vi "WILT Index Station Stats.vi"(0 "Station Number":u32, 1 "Cool Down Period (seconds)":dbl[](array[numeric]), 2 "Drying Time (Min)":dbl[](array[numeric]), 3 "Previous Run Statistics":T1[](array[typedef]), 4 "Enable Start Retry in":bool[](array[boolean]), 5 "Error In":errorcluster) -> (14 "Station Array Index":u32, 15 "Station Cool Down Period (Sec)":dbl, 16 "Station Drying Time (Min)":dbl, 17 "Previous Cycle Time (Minutes)":dbl, 18 "Enable Start Retry out":bool, 19 "Error Out":errorcluster)   [LabVIEW 2016]
uses:
  Type Definitions/WILT Summary Data.ctl
panel:
  # "Get The Info Associated with the desired station"
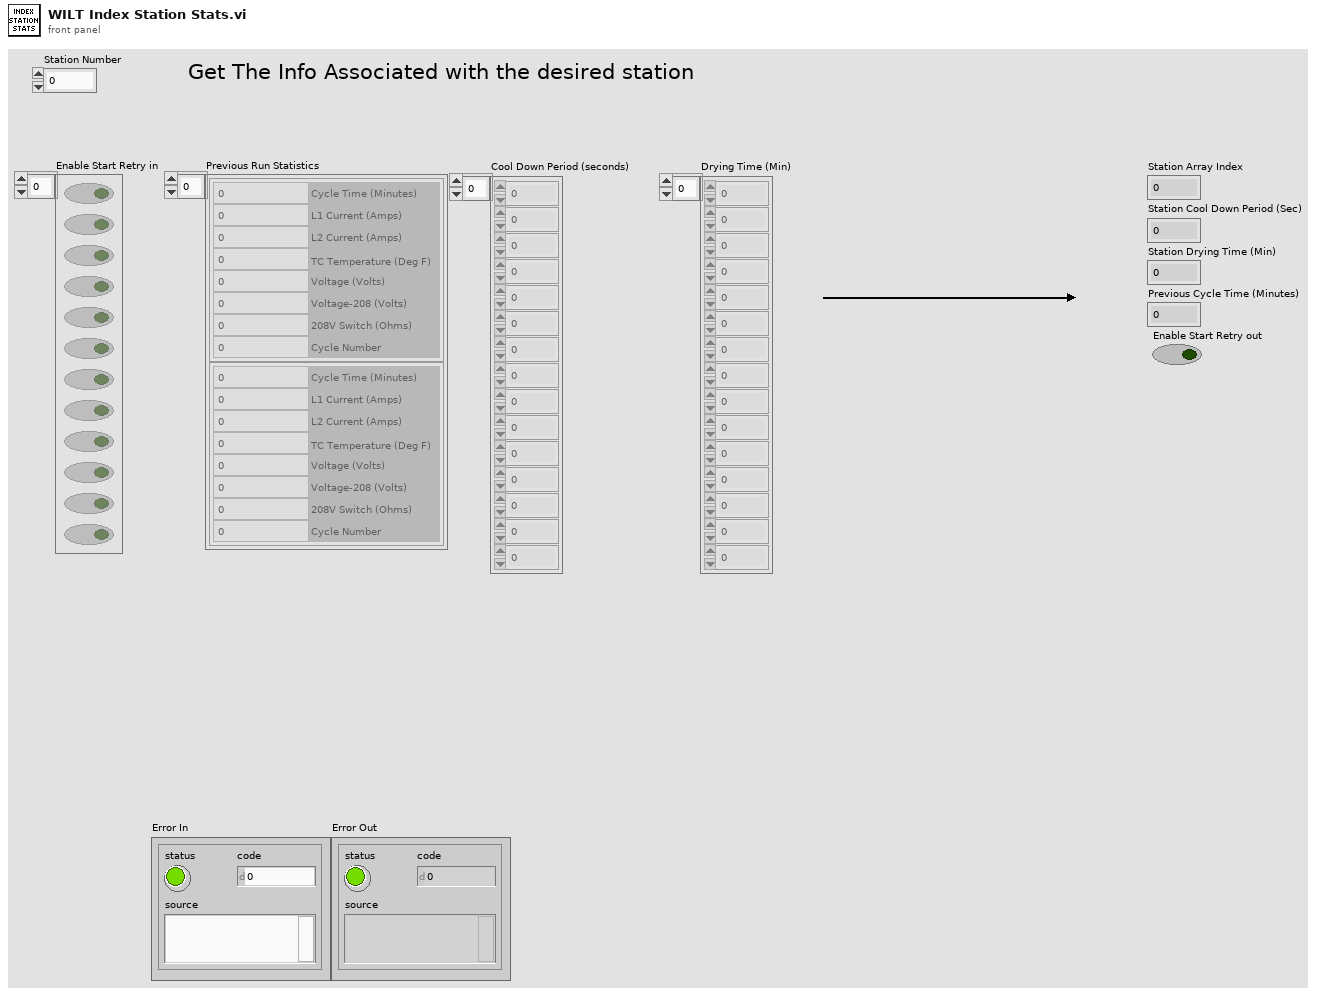
[diagram p1: front panel]
types:
  T1 = typedef "WILT Summary Data.ctl" = cluster{"Cycle Time (Minutes)":dbl, "L1 Current (Amps)":dbl, "L2 Current (Amps)":dbl, "TC Temperature (Deg F)":dbl, "Voltage (Volts)":dbl, "Voltage-208 (Volts)":dbl, "208V Switch (Ohms)":dbl, "Cycle Number":i32}
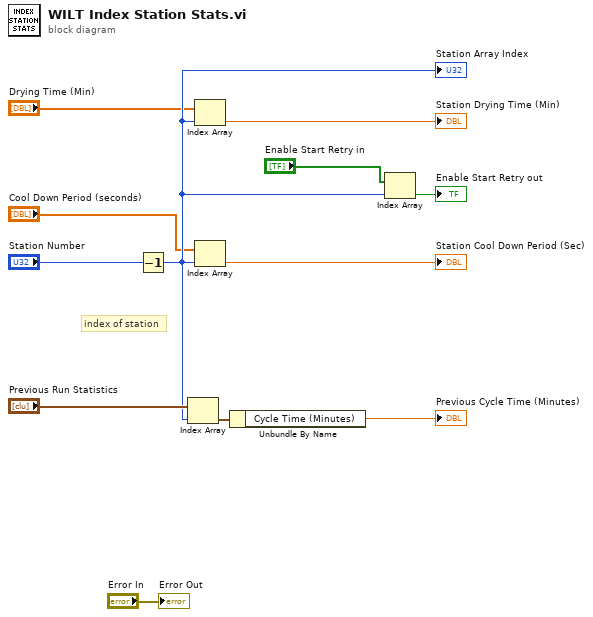
[diagram p0: block diagram]
diagram:
  # "index of station"
  n1 = Decrement(x="Station Number") -> (x-1=w6:u32)
  "Station Array Index" <- w6
  n2 = Index Array(array="Previous Run Statistics", index=w6) -> (element=w12:T1)
  n3 = Index Array(array="Drying Time (Min)", index=w6) -> (element=→"Station Drying Time (Min)":dbl)
  n4 = Index Array(array="Cool Down Period (seconds)", index=w6) -> (element=→"Station Cool Down Period (Sec)":dbl)
  n5 = Unbundle By Name(w12) -> ("Cycle Time (Minutes)"=→"Previous Cycle Time (Minutes)":dbl)
  n6 = Index Array(array="Enable Start Retry in", index=w6) -> (element=→"Enable Start Retry out":bool)
  "Error Out" <- "Error In"
